vi "INWait_Name.vi"(0 "FlowCtrl in":refnum<class "Station Action.lvclass">, 1 "Input2":T1, 5 "Input":T2, 7 "Status":bool=TRUE, 9 "Wait?":bool=TRUE, 11 "error in (no error)":errorcluster, 13 "time(0.1)":i32=100) -> (4 "FlowCtrl out":refnum<class "Station Action.lvclass">, 6 "StatusOut":bool, 8 "TimeOut":bool, 15 "error out":errorcluster)   [LabVIEW 2019]
uses:
  Station Action.lvclass
  FlowCtrl Class/Ctrl/Auto Inspection_IN Name.ctl
  FlowCtrl Class/Ctrl/Auto Inspection_IN Name2.ctl
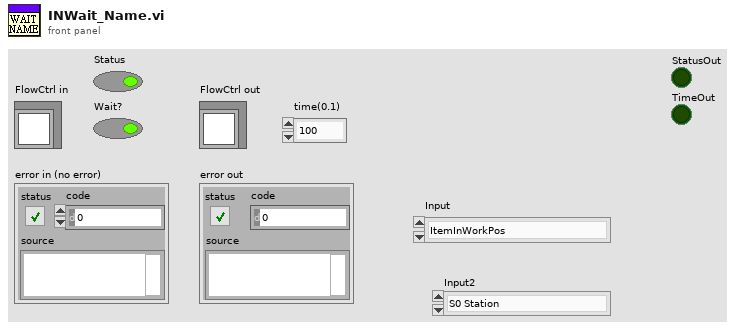
[diagram p1: front panel]
types:
  T1 = typedef "Auto Inspection_IN Name2.ctl" = enum16{"S0 Station", "S1 Barcode ", "S2 Tool Format", "S3 Tool Prpgram", "S4 Tool Sacn", "S11 Laser Detect", "S8 Vision AI"}
  T2 = typedef "Auto Inspection_IN Name.ctl" = enum16{"ItemInWorkPos", "ItemReadyIn", "ItemInSensor", "StopUpSensor", "SlowSensor", "TrayUp", "Fix", "Release fix", "TrayDown", "NextRequest", "StopDown", "ConveyorOut"}
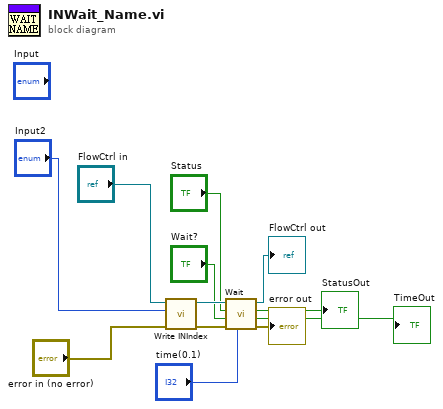
[diagram p0: block diagram]
diagram:
  n1 = call-dynamic "Write INIndex.vi"("error in (no error)"="error in (no error)", "INIndex"="Input2", "Station Action in"="FlowCtrl in") -> ("error out"=w8:errorcluster, "Station Action out"=w7:refnum<class "Station Action.lvclass">)  [unwired: 7 in]
  n2 = call-dynamic "Wait.vi"("time(0.1)"="time(0.1)", "error in (no error)"=w8, "Wait?"="Wait?", "Status"="Status", "FlowCtrl in"=w7) -> ("error out"=→"error out":errorcluster, "TimeOut"=→"TimeOut":bool, "StatusOut"=→"StatusOut":bool, "FlowCtrl out"=→"FlowCtrl out":refnum<class "Station Action.lvclass">)  [unwired: 3 in]
